vi "Graph RT Test Panel.vi"() -> ()   [LabVIEW 2021]
uses:
  Display/Display Manager.lvclass
  Display Utilities/Public/Controls/2D Coordinates.ctl
  Display Utilities/Display Utilities.lvlib
  Display Utilities/Public/Controls/2D Dimensions.ctl
  <vilib>/rvi/interface/nirviCloseFPGA/nirviCloseFPGA.xnode
  <vilib>/rvi/interface/nirviOpenFPGA/nirviOpenFPGA.xnode
  Display/Public/Controls/RGB Gains.ctl
  Graph/Graph.lvclass
  FPGA Bitfiles/Test Neopixel.lvbitx
  <vilib>/FPGAPlugInAG/Dynamic/niLvFpga_Close_Dynamic.vi
  <vilib>/FPGAPlugInAG/myRIO-1900/niLvFpga_Open_myRIO-1900.vi
  <vilib>/rvi/interface/common/dynamic/niFpgaDynamicAddResources.vi
  C:/Git/MEMOSFET/myRIO-Neopixel/Source/RT/Display Element/Display Element.lvclass
  C:/Git/MEMOSFET/myRIO-Neopixel/Source/RT/Graph/Graph.lvclass
  Graph/Public/Controls/Range.ctl
  Graph/Public/Controls/Fill To.ctl
panel:
  in  "period":dbl=0.5
  in  "Update delay":u32=50
  in  "Width G":u32=24 caption="Width"
  in  "Height G":u32=8 caption="Height"
  in  "Fill To":T1
  in  "Range":T2={"Maximum"=2.0, "Minimum"=0.0}
  in  "Intensity":sgl(slide)=0.5 scale=0.0..1.0
  out "Error Out":errorcluster
  in  "FPS":u32(slide)=71 scale=0.0..100.0
  in  "Display X":i32=24 caption="X"
  in  "Display Y":i32=8 caption="Y"
  in  "Position X":i32 caption="X"
  in  "Position Y":i32 caption="Y"
  in  "Force X":i32 caption="X"
  in  "Force Y":i32 caption="Y"
  in  "Layer":u32
  in  "Delete If Outside Bounds":bool=TRUE
  in  "Color":u32(colorbox)=65282
  out "Frame":u32[][](array[colorbox])=[[0, 0, 0, 65282, 65282, 65282, 0, 0, 0, 0, 0, 0, 0, 0, 0, 65282, 65282, 65282, 0, 0, 0, 0, 0, 0], [0, 0, 65282, 0, 0, 0, 0, 0, 0, 0, 0, 0, 0, 0, 0, 0, 0, 0, 65282, 0, 0, 0, 0, 0], [0, 0, 0, 0, 0, 0, 65282, 0, 0, 0, 0, 0, 0, 0, 65282, 0, 0, 0, 0, 65282, 0, 0, 0, 0], [0, 65282, 0, 0, 0, 0, 0, 0, 0, 0, 0, 0, 0, 0, 0, 0, 0, 0, 0, 0, 0, 0, 0, 0], [0, 0, 0, 0, 0, 0, 0, 65282, 0, 0, 0, 0, 0, 65282, 0, 0, 0, 0, 0, 0, 65282, 0, 0, 0], [65282, 0, 0, 0, 0, 0, 0, 0, 0, 0, 0, 0, 0, 0, 0, 0, 0, 0, 0, 0, 0, 0, 0, 0], [0, 0, 0, 0, 0, 0, 0, 0, 65282, 0, 0, 0, 65282, 0, 0, 0, 0, 0, 0, 0, 0, 65282, 0, 0], [0, 0, 0, 0, 0, 0, 0, 0, 0, 65282, 65282, 65282, 0, 0, 0, 0, 0, 0, 0, 0, 0, 0, 65282, 65282]]
  in  "stop":bool
  # "Display Settings"
  # "Display Size"
  # "Display Elements Creation"
  # "Display Elements Properties"
  # "Position"
  # "Force"
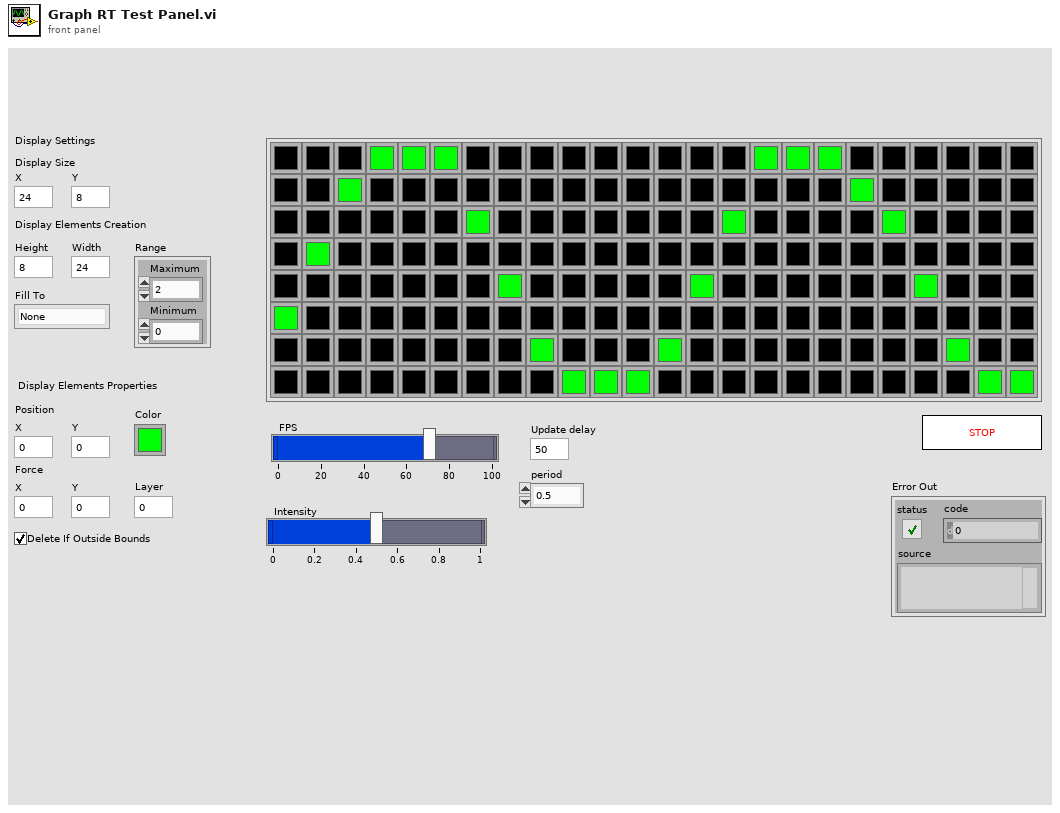
[diagram p1: front panel]
types:
  T1 = typedef "Graph.lvclass/Fill To.ctl" = enum16{"None", "Inf", "-Inf"}
  T2 = typedef "Graph.lvclass/Range.ctl" = cluster{"Maximum":dbl, "Minimum":dbl}
  T3 = typedef "Display Utilities.lvlib/2D Dimensions.ctl" = cluster{"Width":i32, "Height":i32}
  T4 = typedef "RGB Gains.ctl" = cluster{"Red":sgl, "Green":sgl, "Blue":sgl}
  T5 = typedef "Display Utilities.lvlib/2D Coordinates.ctl" = cluster{"X":i32, "Y":i32}
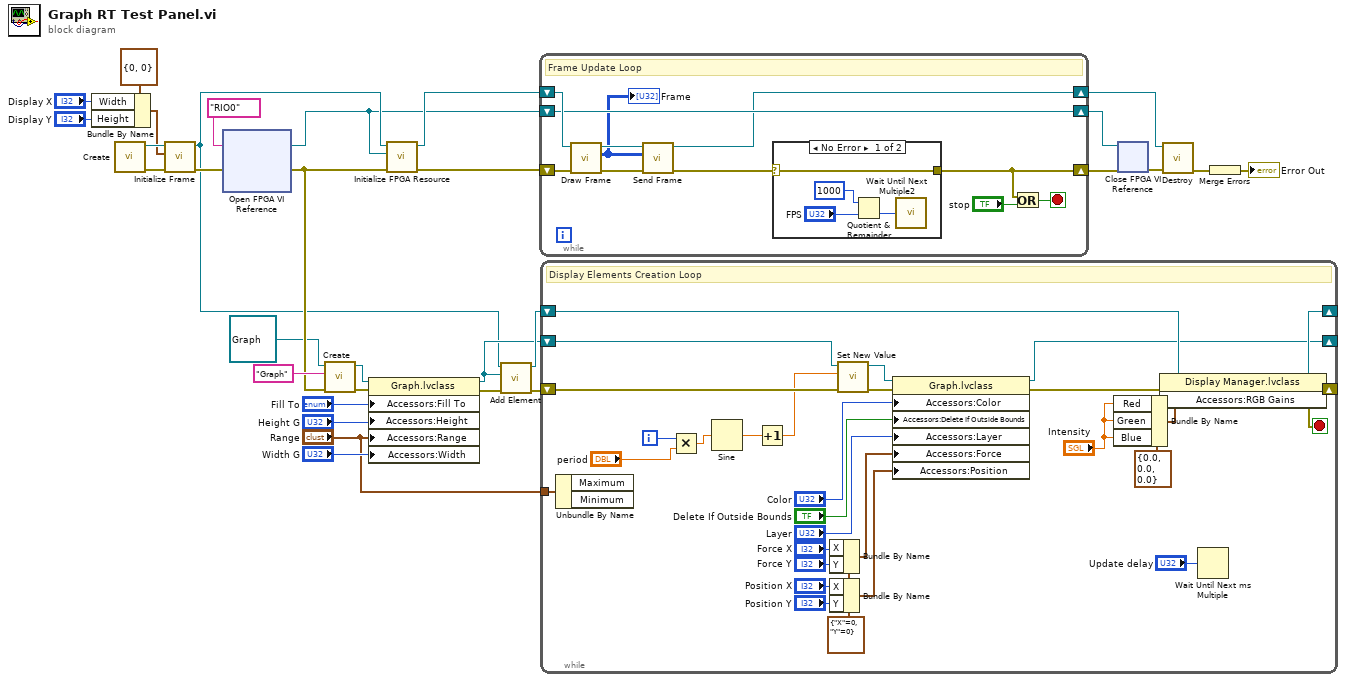
[diagram p0: block diagram]
diagram:
  n1 = Bundle By Name(cluster=T3 {"Width"=0, "Height"=0} ("Size"), "Width"="Display X", "Height"="Display Y") -> (w26:T3)
  n2 = call "Create.vi"() -> ("Error Out"=w30:errorcluster, "Display Manager Out"=w31:refnum<class "Display Manager.lvclass">)  [unwired: 10 in]
  n3 = call "Initialize Frame.vi"("Error In"=w30, "Size"=w26, "Display Manager In"=w31) -> ("Error Out"=w24:errorcluster, "Display Manager Out"=w5:refnum<class "Display Manager.lvclass">)  [unwired: 7 in]
  n4 = xnode "Open FPGA VI Reference"("error in"=w24, "resource name"=tag "RIO0") -> ("FPGA VI Reference Out"=w3:refnum<k20>, "error out"=w6:errorcluster)
  n5 = call-dynamic "Create.vi"("Error In"=w6, "Tag"="Graph", "Graph In"=refnum<class "Graph.lvclass"> refnum ("Graph.lvclass")) -> ("Error Out"=w19:errorcluster, "Graph Out"=w18:refnum<class "Graph.lvclass">)  [unwired: 7 in]
  n6 = property class="Graph.lvclass"(reference=w18, error in=w19, "Accessors:Fill To"="Fill To", "Accessors:Height"="Height G", "Accessors:Range"="Range", "Accessors:Width"="Width G") -> (reference out=w11:refnum<class "Graph.lvclass">, error out=w13:errorcluster)
  n7 = call "Initialize FPGA Resource.vi"("Error In"=w6, "FPGA VI Reference"=w3, "Display In"=w5) -> ("Error Out"=w2:errorcluster, "Display Out"=w4:refnum<class "Display Manager.lvclass">)  [unwired: 7 in]
  n8 = call "Add Element.vi"("Error In"=w13, "New Element"=w11, "Display Manager In"=w5) -> ("Error Out"=w12:errorcluster, "Display Manager Out"=w14:refnum<class "Display Manager.lvclass">)  [unwired: 7 in]
  n9 = while {
    shift-right: [w38] -> w7
    shift-left: w2 -> [w41]
    shift-right: [w32] -> w9
    shift-left: w4 -> [w40]
    shift-right: [w39] -> w8
    shift-left: w3 -> [w39]
    stop <- w42 stop-if-true
    # "Frame Update Loop"
    n10 = call "Draw Frame.vi"("Error In"=w41, "Display Manager In"=w40) -> ("Error Out"=w35:errorcluster, "Frame"=w34:u32[][], "Display Manager Out"=w36:refnum<class "Display Manager.lvclass">)  [unwired: 7 in]
    "Frame" <- w34
    n11 = call "Send Frame.vi"("Error In"=w35, "Frame"=w34, "Display In"=w36) -> ("Error Out"=w33:errorcluster, "Display Out"=w32:refnum<class "Display Manager.lvclass">)  [unwired: 7 in]
    n12 = case shown="No Error" w33 {
      selector: w33 -> [w44 w47]
      tunnel: [w44 w47] -> w38
      frame No Error {
        n13 = Quotient & Remainder(x=u32 1000 ("y"), y="FPS") -> (floor(x/y)=w46:u32)  [unwired: 1 out]
        n14 = call "Wait Until Next Multiple2"("Count(mSec)"=w46) -> ()  [unwired: 1 out]
      }
      frame Error {
      }
    }
    n15 = Or(x=w38, y="stop") -> (x .or. y?=w42:bool)
  }
  n16 = while {
    shift-right: [w71] -> _
    shift-left: w14 -> [w72]
    shift-right: [w70] -> _
    shift-left: w12 -> [w53]
    shift-right: [w68] -> _
    shift-left: w11 -> [w69]
    tunnel: "Range" -> [w54]
    i -> [w50]
    stop <- w70 stop-if-true
    w63 = T5 {"X"=0, "Y"=0} ("Force")
    # "Display Elements Creation Loop"
    n17 = Unbundle By Name(w54) -> ()  [unwired: 2 out]
    n18 = Multiply(x=w50, y="period") -> (x*y=w49:dbl)
    n19 = Sine(x=w49) -> (sin(x)=w52:dbl)
    n20 = Increment(x=w52) -> (x+1=w51:dbl)
    n21 = Bundle By Name(cluster=w63, "X"="Force X", "Y"="Force Y") -> (w62:T5)
    n22 = Bundle By Name(cluster=w63, "X"="Position X", "Y"="Position Y") -> (w61:T5)
    n23 = call "Set New Value.vi"("Error In"=w53, "New Value"=w51, "Graph In"=w69) -> ("Error Out"=w55:errorcluster, "Graph Out"=w56:refnum<class "Graph.lvclass">)  [unwired: 7 in]
    n24 = property class="Graph.lvclass"(reference=w56, error in=w55, "Accessors:Color"="Color", "Accessors:Delete If Outside Bounds"="Delete If Outside Bounds", "Accessors:Layer"="Layer", "Accessors:Force"=w62, "Accessors:Position"=w61) -> (reference out=w68:refnum<class "Graph.lvclass">, error out=w73:errorcluster)
    n25 = Bundle By Name(cluster=T4 {"Red"=0.0, "Green"=0.0, "Blue"=0.0} ("RGB Gains"), "Red"="Intensity", "Green"="Intensity", "Blue"="Intensity") -> (w76:T4)
    n26 = property class="Display Manager.lvclass"(reference=w72, error in=w73, "Accessors:RGB Gains"=w76) -> (reference out=w71:refnum<class "Display Manager.lvclass">, error out=w70:errorcluster)
    n27 = Wait Until Next ms Multiple(millisecond multiple="Update delay") -> ()  [unwired: 1 out]
  }
  n28 = xnode "Close FPGA VI Reference"("FPGA VI Reference In"=w8, "error in"=w7) -> ("error out"=w23:errorcluster)
  n29 = call "Destroy.vi"("Error In"=w23, "Display Manager In"=w9) -> ("Error Out"=w22:errorcluster)  [unwired: 9 in]
  n30 = Merge Errors(w22) -> (→"Error Out":errorcluster)
